vi "server.vi"() -> ()   [LabVIEW 2016]
panel:
  in  "Stop":bool
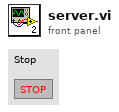
[diagram p1: front panel]
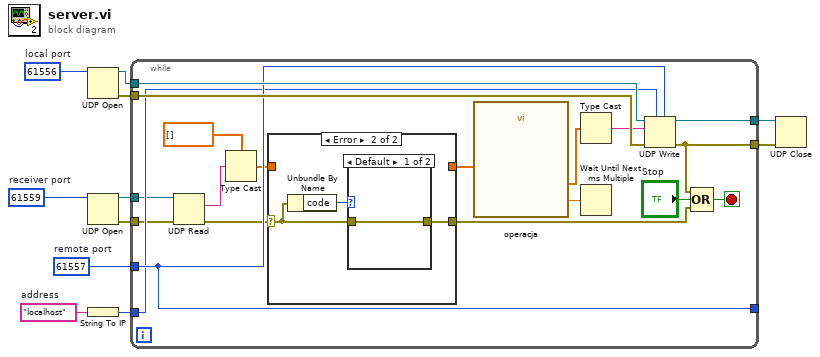
[diagram p0: block diagram]
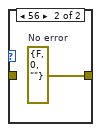
[diagram p3: hidden frame]
diagram:
  w2 = u16 61559  # receiver port
  w7 = u16 61557  # remote port
  w10 = u16 61556  # local port
  w11 = "localhost"  # address
  n1 = UDP Open(11:w10) -> (port=w8:refnum<k16>, 0:w6:errorcluster)  [unwired: 4 in, 1 out]
  n2 = UDP Open(11:w2) -> (port=w1:refnum<k16>, 0:w3:errorcluster)  [unwired: 4 in, 1 out]
  n3 = String To IP(1:w11) -> (0:w9:u32)
  n4 = while {
    tunnel: w9 -> [w21]
    tunnel: w8 -> [w25]
    tunnel: [w24] -> _
    tunnel: w7 -> [w24]
    tunnel: w6 -> [w30]
    tunnel: [w26] -> w5
    tunnel: [w22] -> w4
    tunnel: w3 -> [w15]
    tunnel: w1 -> [w16]
    stop <- w27 stop-if-true
    n5 = UDP Read(connection ID=w16, 8:w15) -> (data out=w19:string, error out=w20:errorcluster)  [unwired: 1 in, 4 out]
    n6 = Type Cast(type=dbl[] [], x=w19) -> (*(type *) &x=w18:dbl[])
    n7 = case shown="Error" w20 {
      selector: w20 -> [w32 w33]
      tunnel: w18 -> [w31 _]
      tunnel: [w32 w34] -> w14
      tunnel: [w31 _] -> w13
      frame No Error {
      }
      frame Error {
        n8 = Unbundle By Name(w33) -> ("code"=w35:i32)
        n9 = case shown="Default" w35 {
          tunnel: [w36 w37] -> w34
          tunnel: w33 -> [w36 _]
          frame Default {
          }
          frame 56 {
            w37 = errorcluster {"status"=FALSE, "code"=0, "source"=""}  # No error
          }
        }
      }
    }
    n10 = call "operacja.vi"("Array in"=w13) -> ("Array out"=w29:dbl[], "Numeric"=w12:dbl)  [unwired: 9 in]
    n11 = Type Cast(x=w29) -> (*(type *) &x=w23:string)  [unwired: 1 out]
    n12 = Wait Until Next ms Multiple(millisecond multiple=w12) -> ()  [unwired: 1 out]
    n13 = UDP Write(address=w21, port or service name=w24, connection ID=w25, data in=w23, 8:w30) -> (error out=w26:errorcluster, 3:w22:refnum<k16>)  [unwired: 1 in]
    n14 = Compound Arithmetic op=OR(w26, "Stop", w14) -> (w27:bool)
  }
  n15 = UDP Close(connection ID=w4, 8:w5) -> ()  [unwired: 2 out]
